vi "save uncaging overlay.vi"(9 "Pixel Coordinates":cluster{"X":u32, "Y":u32}[](array[cluster]), 10 "Image":T2, 11 "param cluster":T1) -> (2 "stripped path":path, 3 "filename without extension":string)   [LabVIEW 2012]
doc: "SciScan 1.0 151216"
uses:
  <vilib>/vision/Image Controls.llb/IMAQ Image.ctl
  <vilib>/Utility/file.llb/Write To Spreadsheet File (I64).vi
panel:
  out "String":string
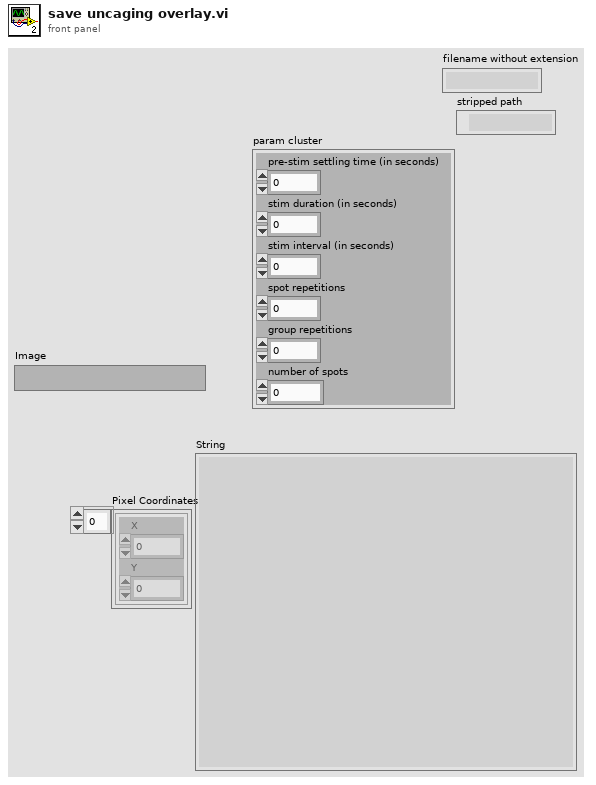
[diagram p1: front panel]
types:
  T1 = cluster{"pre-stim settling time (in seconds)":dbl, "stim duration (in seconds)":dbl, "stim interval (in seconds)":dbl, "spot repetitions":dbl, "group repetitions":dbl, "number of spots":dbl}
  T2 = typedef "IMAQ Image.ctl" = refnum<image>
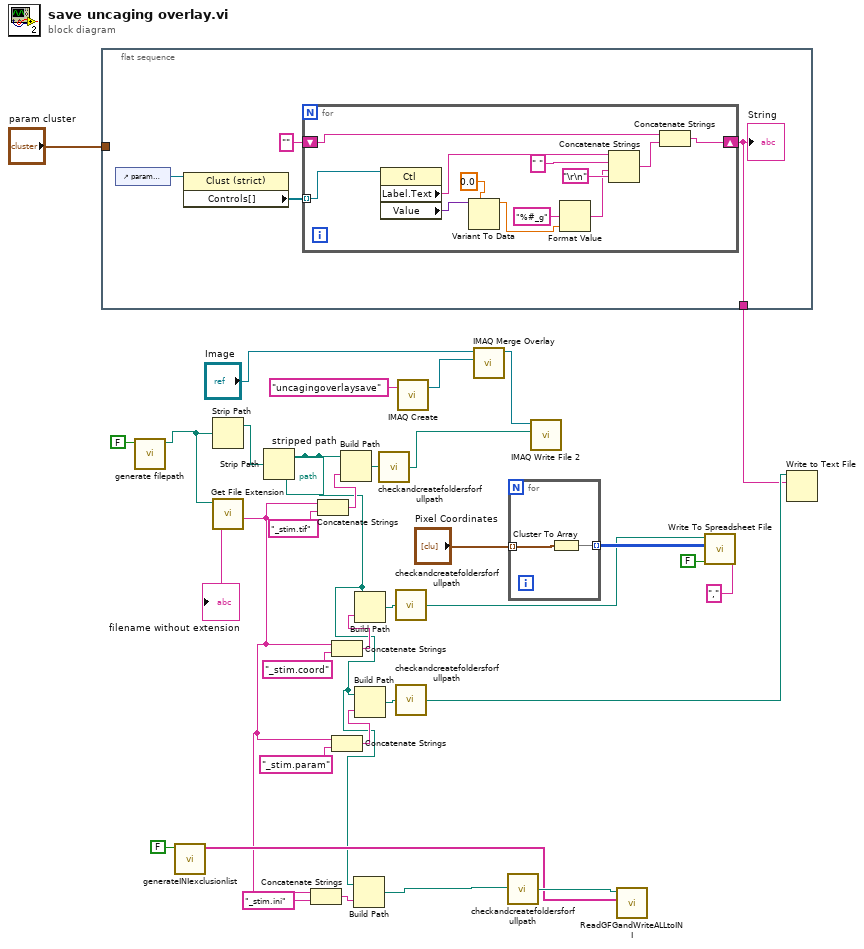
[diagram p0: block diagram]
diagram:
  n1 = flat-sequence {
    tunnel: "param cluster" -> [_]
    tunnel: [w34] -> w13
    frame #0 {
      n2 = control-ref of="param cluster"() -> (w35:refnum<vi>)
      n3 = property class="Clust (strict)"(reference=w35) -> ("Controls[]"=w37:refnum<vi>[])  [unwired: 1 in, 2 out]
      n4 = for {
        tunnel: w37 -> [w49] mode=indexing
        shift-right: [w42] -> w34
        shift-left: "" -> [w41]
        n5 = property class="Ctl"(reference=w49) -> ("Label.Text"=w48:string, "Value"=w46:variant)  [unwired: 1 in, 2 out]
        n6 = Variant To Data(type=0.0, Variant=w46) -> (data=w39:dbl)  [unwired: 1 in, 1 out]
        n7 = Format Value(format string="%#_g", value (0)=w39) -> (output string=w38:string)  [unwired: 1 in]
        n8 = Concatenate Strings(w48, " " ("string"), w38, "\r\n") -> (w43:string)
        n9 = Concatenate Strings(w41, w43) -> (w42:string)
      }
      "String" <- w34
    }
  }
  n10 = call "generate filepath.vi"("set file.path GFG (default: T)"=FALSE) -> ("path"=w33:path)  [unwired: 10 in]
  n11 = call "generateINIexclusionlist.vi"("T for reso, F for galvo"=FALSE) -> ("Array"=w3:string[])  [unwired: 10 in]
  n12 = Strip Path(path=w33) -> (stripped path=w29:path)  [unwired: 1 out]
  n13 = call <vilib>:"Get File Extension.vi"("file"=w33) -> ("filename without extension"=w2:string)  [unwired: 7 in, 3 out]
  "filename without extension" <- w2
  n14 = Strip Path(path=w29) -> (stripped path=w1:path)  [unwired: 1 out]
  "stripped path" <- w1
  n15 = Concatenate Strings(w2, "_stim.ini" ("string")) -> (w5:string)
  n16 = Concatenate Strings(w2, "_stim.tif" ("string")) -> (w32:string)
  n17 = Concatenate Strings(w2, "_stim.coord" ("string")) -> (w24:string)
  n18 = Concatenate Strings(w2, "_stim.param" ("string")) -> (w17:string)
  n19 = Build Path(base path=w1, name or relative path=w32) -> (appended path=w31:path)
  n20 = Build Path(base path=w1, name or relative path=w5) -> (appended path=w7:path)
  n21 = Build Path(base path=w1, name or relative path=w24) -> (appended path=w22:path)
  n22 = Build Path(base path=w1, name or relative path=w17) -> (appended path=w18:path)
  n23 = call "checkandcreatefoldersforfullpath.vi"("Path IN"=w31) -> ("Path OUT"=w30:path)  [unwired: 4 in]
  n24 = call "checkandcreatefoldersforfullpath.vi"("Path IN"=w22) -> ("Path OUT"=w21:path)  [unwired: 4 in]
  n25 = call "checkandcreatefoldersforfullpath.vi"("Path IN"=w18) -> ("Path OUT"=w14:path)  [unwired: 4 in]
  n26 = call "IMAQ Create"("Image Name"="uncagingoverlaysave") -> ("New Image"=w11:T2)  [unwired: 4 in, 1 out]
  n27 = call "IMAQ Merge Overlay"("Image Dst"=w11, "Image Src"="Image") -> ("Image Dst Out"=w9:T2)  [unwired: 8 in, 1 out]
  n28 = call "checkandcreatefoldersforfullpath.vi"("Path IN"=w7) -> ("Path OUT"=w4:path)  [unwired: 4 in]
  n29 = for {
    tunnel: "Pixel Coordinates" -> [w51] mode=indexing
    tunnel: [w50] -> w26 mode=indexing
    n30 = Cluster To Array(cluster=w51) -> (array=w50:u32[])
  }
  n31 = call-poly "IMAQ Write File 2"("File Path"=w30, "Image"=w9) -> ()  [unwired: 8 in, 2 out]
  n32 = call "ReadGFGandWriteALLtoINI.vi"("exclusion regexp array"=w3, "Path"=w4) -> ()  [unwired: 9 in, 1 out]
  n33 = call-poly <vilib>:"Write To Spreadsheet File.vi"("delimiter (\\t)"="," ("delimiter (\\t)"), "append to file? (new file:F)"=FALSE, "2D data"=w26, "file path (dialog if empty)"=w21) -> ()  [unwired: 4 in, 1 out]
  n34 = Write to Text File(file (use dialog)=w14, text=w13) -> ()  [unwired: 2 in, 3 out]
